vi "ziModStart.vi"(8 "Error In":errorcluster, 9 "module Id":T1 items=["sweep", "scopeModule", "dataAcquisitionModule", "pidAdvisor", "awgModule", "impedanceModule", "multiDeviceSyncModule", "zoomFFT", "trigger", "deviceSettings", "record", "precompensationAdvisor"], 11 "Handle In":T3 {"Handle" format="0x%08x"; "Conn" format="0x%08x"}) -> (0 "Error Out":errorcluster, 2 "ModHandle Out":T2 {"ModHandle" format="0x%08x"; "Conn" format="0x%08x"}, 3 "Handle Out":T3 {"Handle" format="0x%08x"; "Conn" format="0x%08x"})   [LabVIEW 2018, in "Zurich Instruments LabOne.lvlib"]
doc: "Creates a module. module Id allows to select following modules: sweep, zoomFFT, record, plladvisor, pidadvisor. \n\nFrom the Handle a ModHandle is created. If the Handle is closed also all corresponding ModHandle are closed."
uses:
  Zurich Instruments LabOne.lvlib
  ziTypeModHandle.ctl
  <instrlib>/Zurich Instruments LabOne/Private/ziLV64.framework
  ziTypeHandle.ctl
  ziTypeModEnum.ctl
panel:
  # "\"sweep\", \n\"zoomFFT\",\n\"trigger\",\n\"deviceSettings\", \n\"record\",\n\"pllAdvisor\",\n\"pidAdvisor\""
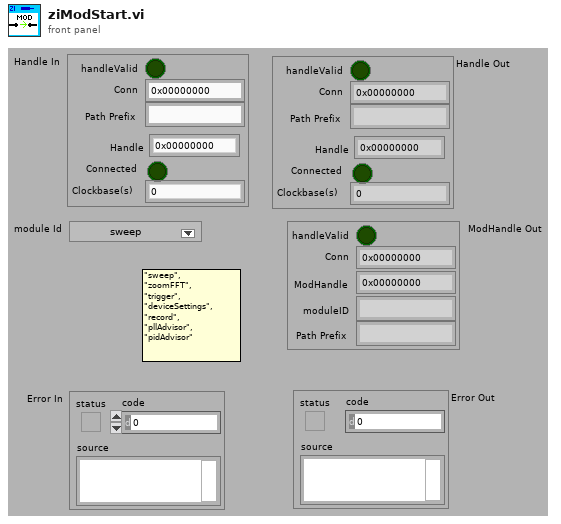
[diagram p1: front panel]
types:
  T1 = typedef "Zurich Instruments LabOne.lvlib/ziTypeModEnum.ctl" = u16
  T2 = typedef "Zurich Instruments LabOne.lvlib/ziTypeModHandle.ctl" = cluster{"handleValid":bool, "Conn":u64, "ModHandle":u64, "moduleID":string, "Path Prefix":string}
  T3 = typedef "Zurich Instruments LabOne.lvlib/ziTypeHandle.ctl" = cluster{"handleValid":bool, "Conn":u64, "Path Prefix":string, "Handle":u64, "Connected":bool, "Clockbase(s)":dbl}
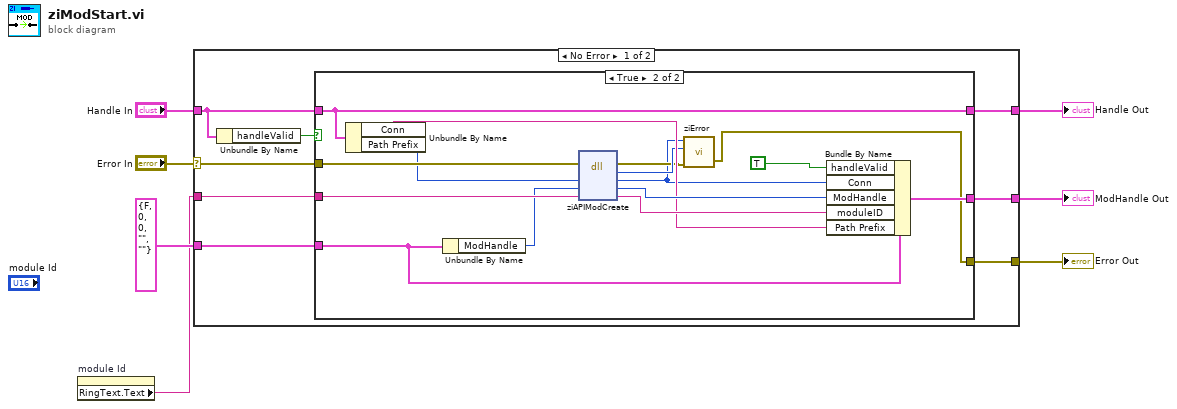
[diagram p0: block diagram]
diagram:
  n1 = property on="module Id" class="Ring (strict)"() -> ("RingText.Text"=w1:string)  [unwired: 2 in, 2 out]
  n2 = case shown="No Error" "Error In" {
    selector: "Error In" -> [w13 w36]
    tunnel: "Handle In" -> [w11 w35]
    tunnel: [w15 w35] -> w6
    tunnel: [w14 w36] -> w5
    tunnel: [w12 w34] -> w3
    tunnel: w1 -> [w9 _]
    tunnel: T2 {"handleValid"=FALSE, "Conn"=0, "ModHandle"=0, "moduleID"="", "Path Prefix"=""} ("ziModHandle") -> [w8 w34]
    frame No Error {
      n3 = Unbundle By Name(w11) -> ("handleValid"=w10:bool)
      n4 = case shown="True" w10 {
        tunnel: w11 -> [w18 w24]
        tunnel: [w18 w24] -> w15
        tunnel: w13 -> [w17 w33]
        tunnel: [w17 w20] -> w14
        tunnel: [w16 w32] -> w12
        tunnel: w9 -> [_ w30]
        tunnel: w8 -> [w16 w27]
        frame False {
        }
        frame True {
          n5 = Unbundle By Name(w24) -> ("Conn"=w25:u64, "Path Prefix"=w23:string)
          n6 = Unbundle By Name(w27) -> ("ModHandle"=w26:u64)
          n7 = dll-call lib="Applications/National Instruments/LabVIEW 2019 64-bit/instr.lib/Zurich Instruments LabOne/Private/ziLV*.*" fn="ziAPIModCreate"(error in=w33, "conn"=w25, "ModHandle"=w26, "moduleId"=w30) -> (error out=w21:errorcluster, "return type"=w22:u32, "conn"=w19:u64, "ModHandle"=w28:u64, "moduleId"=w29:string)  [unwired: 2 in, 1 out]
          n8 = call "ziError.vi"("Conn"=w19, "ziErrorCode"=w22, "Error In"=w21) -> ("Error Out"=w20:errorcluster)  [unwired: 2 in, 1 out]
          n9 = Bundle By Name(cluster=w27, "handleValid"=TRUE, "Conn"=w19, "ModHandle"=w28, "moduleID"=w29, "Path Prefix"=w23) -> (w32:T2)
        }
      }
    }
    frame Error {
    }
  }
  "Handle Out" <- w6
  "Error Out" <- w5
  "ModHandle Out" <- w3
